vi "QR.vi"(8 "error in":errorcluster, 9 "Position":cluster{"X":dbl, "Y":dbl, "Theta":dbl}) -> (0 "error out":errorcluster, 1 "Position Out":cluster{"X":dbl, "Y":dbl, "Theta":dbl}, 2 "Image (duplicate)":T1(plugin-control), 4 "G":i32[][](array[numeric]), 5 "Control Angles":dbl[](array[numeric]), 6 "Found?":bool, 7 "Control Points":cluster{"third_x":i32, "third_y":i32}[](array[cluster]))   [LabVIEW 2018]
uses:
  <vilib>/imath/engines/lvmath/Plug In/_Char/NIMS_CH_character datatype.ctl
  <vilib>/Analysis/coordinate.llb/2D Cartesian Coordinate Rotation (Scalar).vi
  <vilib>/imath/engines/lvmath2/RunTimeEngine/Managers/WorkSpace/UID Generator.vi
  <vilib>/imath/engines/lvmath/Plug In/_Char/NIMS_CH_String to Character Array.vi
  <vilib>/imath/engines/lvmath2/RunTimeEngine/IndexRead/NIMS V(S).vi
  <instcachedir>/0/NIMS V(S)_0488751826AF41519A22953C041130DC.lvgen/NIMS V(S)_0488751826AF41519A22953C041130DC_003.vi
  <vilib>/imath/engines/lvmath2/RunTimeEngine/RunTimeType/NIMS_RunTimeType_From StrictType (excl LVString).vi
  <instcachedir>/0/NIMS_RunTimeType_From StrictType (excl LVString)_E7E34A65C99947108168652BAD14964D.lvgen/NIMS_RunTimeType_From StrictType (excl LVString)_E7E34A65C99947108168652BAD14964D_000.vi
  <vilib>/imathl/engines/lvmath/Functions/Error Handling/Create Error.vi
  <vilib>/imath/engines/lvmath2/RunTimeEngine/LocalVariableDefStatement/MC_LocalVariableDefStatement_Display.vi
  <vilib>/imath/engines/lvmath2/RunTimeEngine/Managers/SymbolTable/Clear UID.vi
  <vilib>/imath/engines/lvmath2/RunTimeEngine/NodeEndStatement/NIMS_NodeEndStatement_Output.vi
  <instcachedir>/0/NIMS_NodeEndStatement_Output_53EC0D466D134D7ABD903AC30B43404B.lvgen/NIMS_NodeEndStatement_Output_53EC0D466D134D7ABD903AC30B43404B_011.vi
  <instcachedir>/0/NIMS_NodeEndStatement_Output_53EC0D466D134D7ABD903AC30B43404B.lvgen/NIMS_NodeEndStatement_Output_53EC0D466D134D7ABD903AC30B43404B_001.vi
  <vilib>/imath/engines/lvmath2/RunTimeEngine/ErrorHandling/NIMS_Finalize Error.vi
  <vilib>/imath/engines/lvmath2/RunTimeEngine/BuiltInFunctions/acos/NIMS_acos(C).vi
  <instcachedir>/0/NIMS_acos(C)_EB9F8BBCD4F84158BAE4AC9B979C42E8.lvgen/NIMS_acos(C)_EB9F8BBCD4F84158BAE4AC9B979C42E8_001.vi
  <vilib>/imath/engines/lvmath2/RunTimeEngine/BuiltInFunctions/round/NIMS_round(DBL-S).vi
  <vilib>/imath/engines/lvmath2/RunTimeSupport/NIMS_Error if Not Equal.vi
  <instcachedir>/0/NIMS_Error if Not Equal_C77461FADD9B4AE6B0EA3ED6E3A6D94D.lvgen/NIMS_Error if Not Equal_C77461FADD9B4AE6B0EA3ED6E3A6D94D_000.vi
  <vilib>/imath/engines/lvmath2/RunTimeEngine/IndexReplace/NIMS M(S,S)=S.vi
  <instcachedir>/0/NIMS M(S,S)=S_5DAF17B45D8A4C8588C7CF468644990A.lvgen/NIMS M(S,S)=S_5DAF17B45D8A4C8588C7CF468644990A_002.vi
  <vilib>/imath/engines/lvmath2/RunTimeEngine/ErrorHandling/NIMS_Create Error From Enums.vi
  <vilib>/imath/engines/lvmath2/RunTimeEngine/RangeToken/NIMS_Range_R2 - Integer.vi
  <instcachedir>/0/NIMS_Range_R2 - Integer_E35B921DECF84AADB7325A02D418BFCC.lvgen/NIMS_Range_R2 - Integer_E35B921DECF84AADB7325A02D418BFCC_000.vi
  <vilib>/imath/engines/lvmath2/RunTimeEngine/CommandStatement/MC_CommandStatement_break.vi
  <vilib>/imath/engines/lvmath2/RunTimeEngine/BuiltInFunctions/min/2 inputs/NIMS_min(RG,RG)-no size check.vi
  <instcachedir>/0/NIMS_min(RG,RG)-no size check_7F67BAB91AFC452D9517D2EA1C8F5F88.lvgen/NIMS_min(RG,RG)-no size check_7F67BAB91AFC452D9517D2EA1C8F5F88_001.vi
  <vilib>/imath/engines/lvmath2/RunTimeEngine/BuiltInFunctions/max/2 inputs/NIMS_max(RG,RG)-no size check.vi
  <instcachedir>/0/NIMS_max(RG,RG)-no size check_F871939977644B7683C1350DCCAD7557.lvgen/NIMS_max(RG,RG)-no size check_F871939977644B7683C1350DCCAD7557_001.vi
  <instcachedir>/0/NIMS_Range_R2 - Integer_E35B921DECF84AADB7325A02D418BFCC.lvgen/NIMS_Range_R2 - Integer_E35B921DECF84AADB7325A02D418BFCC_001.vi
  <vilib>/imath/engines/lvmath2/RunTimeEngine/IndexRead/NIMS M(S,S).vi
  <instcachedir>/0/NIMS M(S,S)_AC51E74150A542F7991B9634C66F3096.lvgen/NIMS M(S,S)_AC51E74150A542F7991B9634C66F3096_002.vi
  <instcachedir>/0/NIMS_min(RG,RG)-no size check_7F67BAB91AFC452D9517D2EA1C8F5F88.lvgen/NIMS_min(RG,RG)-no size check_7F67BAB91AFC452D9517D2EA1C8F5F88_002.vi
  <instcachedir>/0/NIMS_min(RG,RG)-no size check_7F67BAB91AFC452D9517D2EA1C8F5F88.lvgen/NIMS_min(RG,RG)-no size check_7F67BAB91AFC452D9517D2EA1C8F5F88_003.vi
  <instcachedir>/0/NIMS_NodeEndStatement_Output_53EC0D466D134D7ABD903AC30B43404B.lvgen/NIMS_NodeEndStatement_Output_53EC0D466D134D7ABD903AC30B43404B_016.vi
  <vilib>/imath/engines/lvmath2/RunTimeEngine/BuiltInFunctions/mod/NIMS_mod_no_size_check.vi
  <instcachedir>/0/NIMS_mod_no_size_check_5393E3382FD241D281EEB71DA286C65B.lvgen/NIMS_mod_no_size_check_5393E3382FD241D281EEB71DA286C65B_001.vi
  <vilib>/vision/NI_Vision_Development_Module.lvlib
  <vilib>/Analysis/NI_AALPro.lvlib
  <vilib>/imath/engines/lvmath2/RunTimeEngine/Managers/SymbolTable/NIMS_WorkSpace.lvlib
panel:
  out "Data":string
  in  "ROI Descriptor":T2 {"Contours"."Type" items=["No Selection", "Point", "Line", "Rectangle", "Oval", "Polygon", "Freehand Region", "Annulus", "Unused2", "Unused3", "Broken Line", "Freehand Line", "Rotated Rectangle"]}
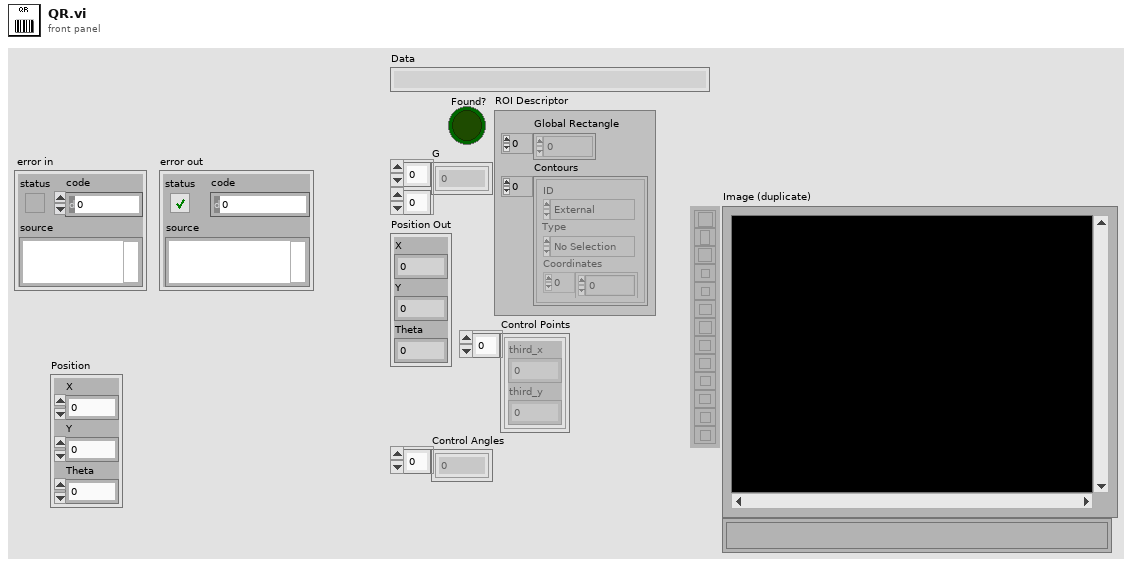
[diagram p1: front panel]
types:
  T1 = typedef "IMAQ Image.ctl" = refnum<image>
  T2 = typedef "ROI Descriptor" = cluster{"Global Rectangle":i32[], "Contours":cluster{"ID":enum32{"External", "Internal"}, "Type":u32, "Coordinates":i32[]}[]}
  T3 = typedef "QR Code Report.ctl" = cluster{"Found?":bool, "Data":string, "Bounding Box":cluster{"x":sgl, "y":sgl}[], "Errors Corrected":u32, "Dimensions (Rows/Cols)":u32, "Version":u32, "QR Model":T4, "Stream Mode":T5, "Barcode Polarity":T6, "Mirrored?":bool, "Append Stream Position":u32, "Size of Append Stream":u32, "First EAN-128 ID":i32, "First Alternate Language ID":i32, "Append Stream ID":u32, "Minimum Edge Strength":u32, "Demodulation Mode":T7, "Cell Sample Size":T8, "Cell Filter Mode":T9}
  T4 = typedef "QR Code Model Type.ctl" = i32
  T5 = typedef "QR Code Stream Mode Type.ctl" = i32
  T6 = typedef "Data Matrix Polarity.ctl" = i32
  T7 = typedef "Demodulation Mode.ctl" = i32
  T8 = typedef "Cell Sample Size.ctl" = i32
  T9 = typedef "Cell Filter Mode.ctl" = i32
  T10 = typedef "NIMS_CH_character datatype.ctl" = cluster{"Numeric":u8}
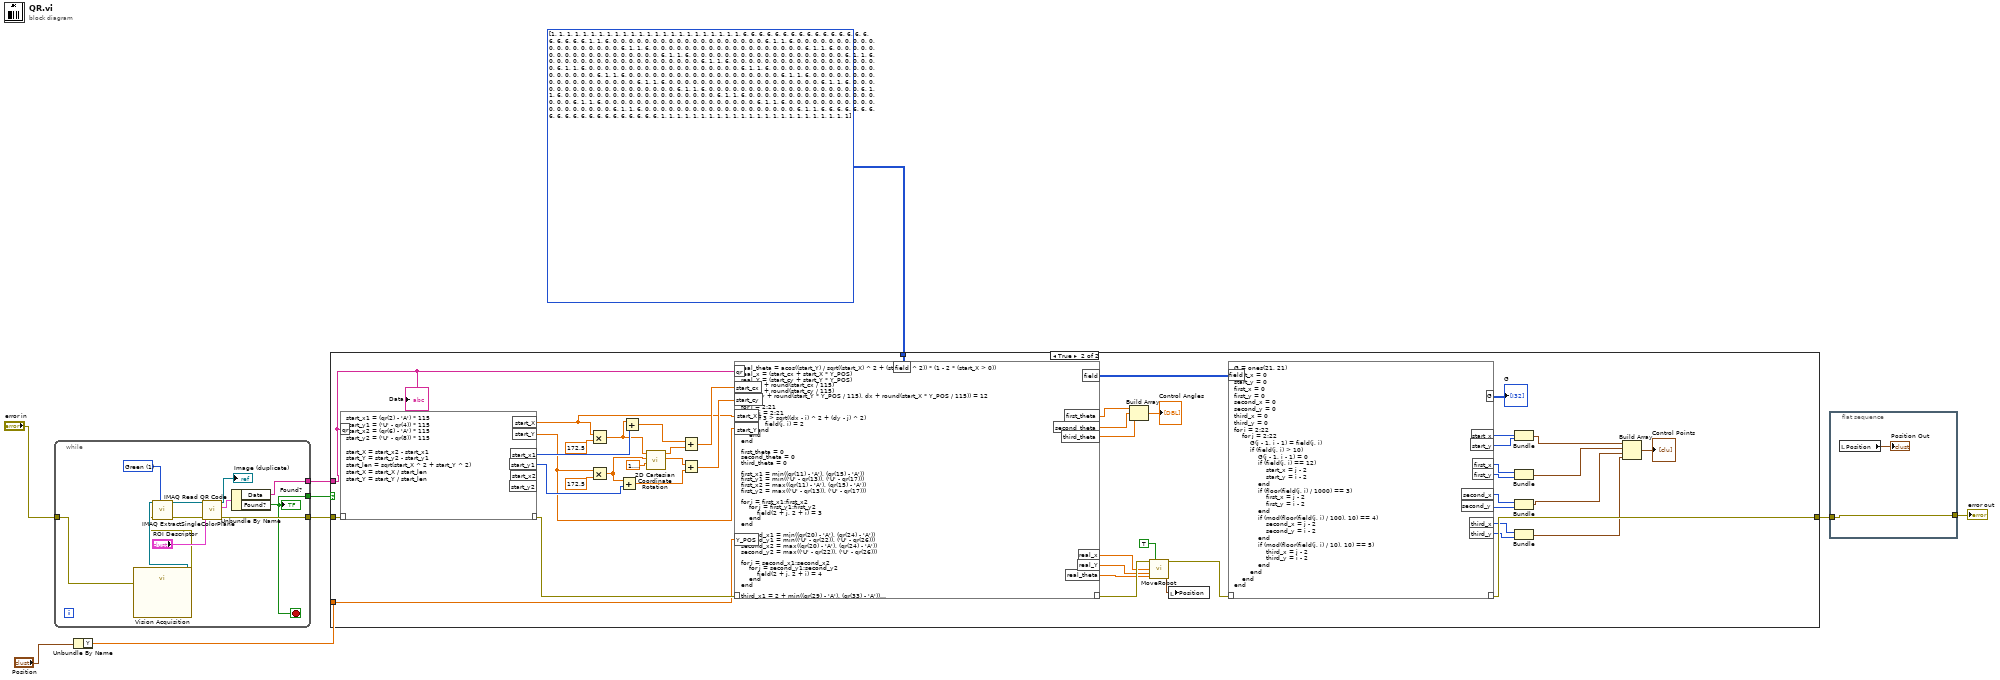
[diagram p0: block diagram]
diagram:
  n1 = while {
    tunnel: [w10] -> w9
    tunnel: [w14] -> w7
    tunnel: "error in" -> [w13]
    tunnel: [w16] -> w8
    stop <- w10 stop-if-true
    w21 = 1 items=["Red", "Green", "Blue", "Hue", "Saturation", "Luminance", "Value", "Intensity"] ("Color Plane")
    n2 = call "Vision Acquisition"("error in"=w13) -> ("Image Out"=w12:T1, "error out"=w11:errorcluster)  [unwired: 25 in]
    n3 = call "IMAQ ExtractSingleColorPlane"("Color Plane"=w21, "error in (no error)"=w11, "Image Src"=w12) -> ("error out"=w20:errorcluster, "Image Dst Out"=w19:T1)  [unwired: 7 in]
    n4 = call "IMAQ Read QR Code"("error in (no error)"=w20, "ROI Descriptor"="ROI Descriptor", "Image"=w19) -> ("error out"=w16:errorcluster, "QR Code Report"=w17:T3, "Image (duplicate)"=→"Image (duplicate)":T1)  [unwired: 5 in, 1 out]
    n5 = Unbundle By Name(w17) -> ("Data"=w14:string, "Found?"=w10:bool)
    "Found?" <- w10
  }
  n6 = Unbundle By Name("Position") -> ("Y"=w6:dbl)
  n7 = case shown="True" w9 {
    tunnel: w8 -> [w22 w69]
    tunnel: w7 -> [_ w55]
    tunnel: [w22 w40] -> w4
    tunnel: w6 -> [_ w51]
    tunnel: u8[][] [[1, 1, 1, 1, 1, 1, 1, 1, 1, 1, 1, 1, 1, 1, 1, 1, 1, 1, 1, 1, 1, 1, 1], [1, 6, 6, 6, 6, 6, 6, 6, 6, 6, 6, 6, 6, 6, 6, 6, 6, 6, 6, 6, 6, 6, 1], [1, 6, 0, 0, 0, 0, 0, 0, 0, 0, 0, 0, 0, 0, 0, 0, 0, 0, 0, 0, 0, 6, 1], [1, 6, 0, 0, 0, 0, 0, 0, 0, 0, 0, 0, 0, 0, 0, 0, 0, 0, 0, 0, 0, 6, 1], [1, 6, 0, 0, 0, 0, 0, 0, 0, 0, 0, 0, 0, 0, 0, 0, 0, 0, 0, 0, 0, 6, 1], [1, 6, 0, 0, 0, 0, 0, 0, 0, 0, 0, 0, 0, 0, 0, 0, 0, 0, 0, 0, 0, 6, 1], [1, 6, 0, 0, 0, 0, 0, 0, 0, 0, 0, 0, 0, 0, 0, 0, 0, 0, 0, 0, 0, 6, 1], [1, 6, 0, 0, 0, 0, 0, 0, 0, 0, 0, 0, 0, 0, 0, 0, 0, 0, 0, 0, 0, 6, 1], [1, 6, 0, 0, 0, 0, 0, 0, 0, 0, 0, 0, 0, 0, 0, 0, 0, 0, 0, 0, 0, 6, 1], [1, 6, 0, 0, 0, 0, 0, 0, 0, 0, 0, 0, 0, 0, 0, 0, 0, 0, 0, 0, 0, 6, 1], [1, 6, 0, 0, 0, 0, 0, 0, 0, 0, 0, 0, 0, 0, 0, 0, 0, 0, 0, 0, 0, 6, 1], [1, 6, 0, 0, 0, 0, 0, 0, 0, 0, 0, 0, 0, 0, 0, 0, 0, 0, 0, 0, 0, 6, 1], [1, 6, 0, 0, 0, 0, 0, 0, 0, 0, 0, 0, 0, 0, 0, 0, 0, 0, 0, 0, 0, 6, 1], [1, 6, 0, 0, 0, 0, 0, 0, 0, 0, 0, 0, 0, 0, 0, 0, 0, 0, 0, 0, 0, 6, 1], [1, 6, 0, 0, 0, 0, 0, 0, 0, 0, 0, 0, 0, 0, 0, 0, 0, 0, 0, 0, 0, 6, 1], [1, 6, 0, 0, 0, 0, 0, 0, 0, 0, 0, 0, 0, 0, 0, 0, 0, 0, 0, 0, 0, 6, 1], [1, 6, 0, 0, 0, 0, 0, 0, 0, 0, 0, 0, 0, 0, 0, 0, 0, 0, 0, 0, 0, 6, 1], [1, 6, 0, 0, 0, 0, 0, 0, 0, 0, 0, 0, 0, 0, 0, 0, 0, 0, 0, 0, 0, 6, 1], [1, 6, 0, 0, 0, 0, 0, 0, 0, 0, 0, 0, 0, 0, 0, 0, 0, 0, 0, 0, 0, 6, 1], [1, 6, 0, 0, 0, 0, 0, 0, 0, 0, 0, 0, 0, 0, 0, 0, 0, 0, 0, 0, 0, 6, 1], [1, 6, 0, 0, 0, 0, 0, 0, 0, 0, 0, 0, 0, 0, 0, 0, 0, 0, 0, 0, 0, 6, 1], [1, 6, 6, 6, 6, 6, 6, 6, 6, 6, 6, 6, 6, 6, 6, 6, 6, 6, 6, 6, 6, 6, 1], [1, 1, 1, 1, 1, 1, 1, 1, 1, 1, 1, 1, 1, 1, 1, 1, 1, 1, 1, 1, 1, 1, 1]] ("Field") -> [_ w50]
    frame False {
    }
    frame True {
      n8 = mathscript code="start_x1 = (qr(2) - 'A') * 115\nstart_y1 = ('U' - qr(4)) * 115\nstart_x2 = (qr(6) - 'A') * 115\nstart_y2 = ('U' - qr(8)) * 115\n\nstart_X = start_x2 - start_x1\nstart_Y = start_y2 - start_y1\nstart_len = sqrt(start_X ^ 2 + start_Y ^ 2)\nstart_X = start_X / start_len\nstart_Y = start_Y / start_len"("??"=w69, "qr"=w55) -> ("??"=w54:errorcluster, "start_X"=w53:dbl, "start_Y"=w52:dbl, "start_x1"=w66:i32, "start_y1"=w65:i32)  [unwired: 2 out]
      n9 = Multiply(x=w53, y=172.5) -> (x*y=w63:dbl)
      n10 = Multiply(x=w52, y=172.5) -> (x*y=w62:dbl)
      n11 = Add(x=w62, y=w65) -> (x+y=w60:dbl)
      n12 = Add(x=w63, y=w66) -> (x+y=w58:dbl)
      n13 = call-poly <vilib>:"2D Cartesian Coordinate Rotation.vi"("theta"=1.5707963267948966, "y"=w62, "x"=w63) -> ("y out"=w61:dbl, "x out"=w59:dbl)  [unwired: 6 in, 1 out]
      n14 = Add(x=w58, y=w59) -> (x+y=w57:dbl)
      n15 = Add(x=w61, y=w60) -> (x+y=w56:dbl)
      n16 = mathscript code="real_theta = acos((start_Y) / sqrt((start_X) ^ 2 + (start_Y) ^ 2)) * (1 - 2 * (start_X > 0))\nreal_x = (start_cx + start_X * Y_POS)\nreal_Y = (start_cy + start_Y * Y_POS)\ndx = 2 + round(start_cx / 115)\ndy = 2 + round(start_cy / 115)\nfield(dy + round(start_Y * Y_POS / 115), dx + round(start_X * Y_POS / 115)) = 12\n\nfor i = 2:21\n    for j = 2:21\n        if 3 > sqrt((dx - i) ^ 2 + (dy - j) ^ 2)\n            field(j, i) = 2\n        end\n    end\nend\n\nfirst_theta = 0\nsecond_theta = 0\nthird_theta = 0\n\nfirst_x1 = min((qr(11) - 'A'), (qr(15) - 'A'))\nfirst_y1 = min(('U' - qr(13)), ('U' - qr(17)))\nfirst_x2 = max((qr(11) - 'A'), (qr(15) - 'A'))\nfirst_y2 = max(('U' - qr(13)), ('U' - qr(17)))\n\nfor i = first_x1:first_x2\n    for j = first_y1:first_y2\n        field(2 + j, 2 + i) = 3\n    end\nend\n\nsecond_x1 = min((qr(20) - 'A'), (qr(24) - 'A'))\nsecond_y1 = min(('U' - qr(22)), ('U' - qr(26)))\nsecond_x2 = max((qr(20) - 'A'), (qr(24) - 'A'))\nsecond_y2 = max(('U' - qr(22)), ('U' - qr(26)))\n\nfor i = second_x1:second_x2\n    for j = second_y1:second_y2\n        field(2 + j, 2 + i) = 4\n    end\nend\n\nthird_x1 = 2 + min((qr(29) - 'A'), (qr(33) - 'A'))\nthird_y1 = 2 +min(('U' - qr(31)), ('U' - qr(35)))\nthird_x2 = 2 + max((qr(29) - 'A'), (qr(33) - 'A'))\nthird_y2 = 2 + max(('U' - qr(31)), ('U' - qr(35)))\n\nfor i = third_x1:third_x2\n    for j = third_y1:third_y2\n        field(2 + j, 2 + i) = 5\n    end\nend\n\nfor i = 2:21\n    for j = 2:21\n        if (field(j, i) < 6)\n            if (field(j, i) > 0)\n                if (field(j - 1, i - 1) == 0)\n                     field(j - 1, i - 1) = 6\n                end\n                if (field(j - 1, i) == 0)\n                     field(j - 1, i) = 6\n                end\n                if (field(j - 1, i + 1) == 0)\n                     field(j - 1, i + 1) = 6\n                end\n                if (field(j, i - 1) == 0)\n                     field(j, i - 1) = 6\n                end\n                if (field(j, i + 1) == 0)\n                     field(j, i + 1) = 6\n                end\n                if (field(j + 1, i - 1) == 0)\n                     field(j + 1, i - 1) = 6\n                end\n                if (field(j + 1, i) == 0)\n                     field(j + 1, i) = 6\n                end\n                if (field(j + 1, i + 1) == 0)\n                     field(j + 1, i + 1) = 6\n                end\n            end\n        end\n    end\nend\n\nf_x1 = first_x1\nf_y1 = first_y1\nf_x2 = 21 - first_x2\nf_y2 = 21 - first_y2\n\nmin_dist = min(f_x1, min(f_x2, min(f_y1, f_y2)))\nif min_dist == f_x1\n    field(2 + f_y1 + 1, 2 + 21 -f_x2 + 2) = 3000\n    first_theta = pi / 2\nend\nif min_dist == f_x2\n    field(2 + f_y1 + 1, 2 + f_x1 - 2) = 3000\n    first_theta = -pi / 2\nend\nif min_dist == f_y1\n    field(2 + 21 - f_y2 + 2, 2 + f_x1 + 1) = 3000\n    first_theta = pi\nend\nif min_dist == f_y2\n    field(2 + f_y1 - 2, 2 + f_x1 + 1) = 3000\n    first_theta = 0\nend\n\ns_x1 = second_x1\ns_y1 = second_y1\ns_x2 = 21 - second_x2\ns_y2 = 21 - second_y2\n\nmin_dist = min(s_x1, min(s_x2, min(s_y1, s_y2)))\nif min_dist == s_x1\n    field(2 + s_y1 + 1, 2 + 21 -s_x2 + 2) = field(2 + s_y1 + 1, 2 + 21 -s_x2 + 2) + 400\n    second_theta = pi / 2\nend\nif min_dist == s_x2\n    field(2 + s_y1 + 1, 2 + s_x1 - 2) = field(2 + s_y1 + 1, 2 + s_x1 - 2) + 400\n    second_theta = -pi / 2\nend\nif min_dist == s_y1\n    field(2 + 21 - s_y2 + 2, 2 + s_x1 + 1) =  field(2 + 21 - s_y2 + 2, 2 + s_x1 + 1) + 400\n    second_theta = pi\nend\nif min_dist == s_y2\n    field(2 + s_y1 - 2, 2 + s_x1 + 1) =  field(2 + s_y1 - 2, 2 + s_x1 + 1) + 400\n    second_theta = 0\nend\n\nt_x1 = third_x1\nt_y1 = third_y1\nt_x2 = 21 - third_x2\nt_y2 = 21 - third_y2\n\nmin_dist = min(t_x1, min(t_x2, min(t_y1, t_y2)))\nif min_dist == t_x1\n    field(2 + t_y1 + 1, 2 + 21 -t_x2 + 2) = field(2 + t_y1 + 1, 2 + 21 -t_x2 + 2) + 50\n    third_theta = pi / 2\nend\nif min_dist == t_x2\n    field(2 + t_y1 + 1, 2 + t_x1 - 2) =  field(2 + t_y1 + 1, 2 + t_x1 - 2) + 50\n    third_theta = -pi / 2\nend\nif min_dist == t_y1\n    field(2 + 21 - t_y2 + 2, 2 + t_x1 + 1) = field(2 + 21 - t_y2 + 2, 2 + t_x1 + 1) + 50\n    third_theta = pi\nend\nif min_dist == f_y2\n    field(2 + t_y1 - 2, 2 + t_x1 + 1) =  field(2 + t_y1 - 2, 2 + t_x1 + 1) + 50\n    third_theta = 0\nend"("??"=w54, "start_cx"=w57, "start_cy"=w56, "qr"=w55, "start_X"=w53, "start_Y"=w52, "Y_POS"=w51, "field"=w50) -> ("??"=w49:errorcluster, "real_theta"=w45:dbl, "real_x"=w47:dbl, "real_Y"=w46:dbl, "first_theta"=w26:dbl, "second_theta"=w25:dbl, "third_theta"=w24:dbl, "field"=w42:i32[][])
      n17 = Build Array(w26, w25, w24) -> (→"Control Angles":dbl[])
      n18 = call "MoveRobot.vi"("Error/Flow In"=w49, "Reset"=TRUE, "x (mm/s)"=w47, "y (mm/s)"=w46, "theta (rad/s)"=w45) -> ("Error/Flow Out"=w43:errorcluster, "Position"=w44:cluster{"X":dbl, "Y":dbl, "Theta":dbl})  [unwired: 9 in]
      n19 = local write "Position"(w44) -> ()
      n20 = mathscript code="G = ones(21, 21)\nstart_x = 0\nstart_y = 0\nfirst_x = 0\nfirst_y = 0\nsecond_x = 0\nsecond_y = 0\nthird_x = 0\nthird_y = 0\nfor i = 2:22\n    for j = 2:22\n        G(j - 1, i - 1) = field(j, i)\n        if (field(j, i) > 10)\n            G(j - 1, i - 1) = 0\n            if (field(j, i) == 12)\n                start_x = j - 2\n                start_y = i - 2\n            end\n            if (floor(field(j, i) / 1000) == 3)\n                first_x = j - 2\n                first_y = i - 2\n            end\n            if (mod(floor(field(j, i) / 100), 10) == 4)\n                second_x = j - 2\n                second_y = i - 2\n            end\n            if (mod(floor(field(j, i) / 10), 10) == 5)\n                third_x = j - 2\n                third_y = i - 2\n            end\n        end\n    end\nend"("??"=w43, "field"=w42) -> ("??"=w40:errorcluster, "start_x"=w39:i32, "start_y"=w38:i32, "first_x"=w37:i32, "first_y"=w36:i32, "second_x"=w35:i32, "second_y"=w34:i32, "third_x"=w33:i32, "third_y"=w32:i32, "G"=→"G":i32[][])
      n21 = Bundle("start_x"=w39, "start_y"=w38) -> (w31:cluster{"start_x":i32, "start_y":i32})  [unwired: 1 in]
      n22 = Bundle("first_x"=w37, "first_y"=w36) -> (w30:cluster{"first_x":i32, "first_y":i32})  [unwired: 1 in]
      n23 = Bundle("second_x"=w35, "second_y"=w34) -> (w29:cluster{"second_x":i32, "second_y":i32})  [unwired: 1 in]
      n24 = Bundle("third_x"=w33, "third_y"=w32) -> (w28:cluster{"third_x":i32, "third_y":i32})  [unwired: 1 in]
      n25 = Build Array(w31, w30, w29, w28) -> (→"Control Points":cluster{"third_x":i32, "third_y":i32}[])
      "Data" <- w55
    }
  }
  n26 = flat-sequence {
    tunnel: w4 -> [w4086]
    tunnel: [w4086] -> w3
    frame #0 {
      n27 = local read "Position"() -> (→"Position Out":cluster{"X":dbl, "Y":dbl, "Theta":dbl})
    }
  }
  "error out" <- w3
